vi "Get grpc_reflection_v1alpha_ListServiceResponse.vi"(8 "error in (no error)":errorcluster, 11 "gRPCid":T1) -> (0 "error out":errorcluster, 2 "package_templatemessage":T2, 3 "gRPCid out":T1)   [LabVIEW 2025, in "reflection_server.lvlib"]
uses:
  reflection_server.lvlib
  grpc_reflection_v1alpha_ListServiceResponse.ctl
  grpc_reflection_v1alpha_ServiceResponse.ctl
  <vilib>/gRPC/LabVIEW gRPC Library/Shared/grpcId.ctl
  grpc_reflection_v1alpha_ListServiceResponse_Flat.ctl
  grpc_reflection_v1alpha_ServiceResponse_Flat.ctl
  2ed25e12-861d-4677-8ead-ace2906b2041.vi
  <vilib>/gRPC/LabVIEW gRPC Library/Shared/TranslateGrpcError.vi
  FlatToRichgrpc_reflection_v1alpha_ServiceResponse.vi
  <vilib>/gRPC/LabVIEW gRPC Library/Server API/Server/Get Server DLL Path.vi
  <vilib>/Utility/error.llb/Error Cluster From Error Code.vi
  <vilib>/gRPC/LabVIEW gRPC Library/grpc-lvsupport-release.lvlib
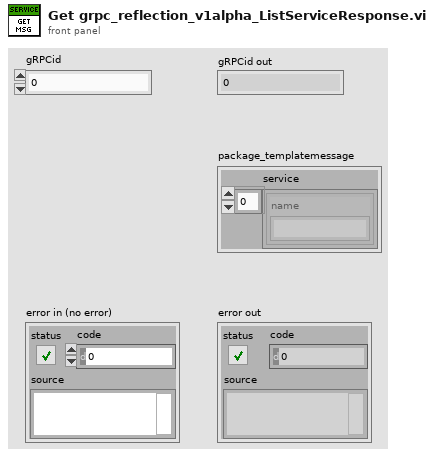
[diagram p1: front panel]
types:
  T1 = typedef "grpc-lvsupport-release.lvlib/grpcId.ctl" = u64
  T2 = typedef "reflection_server.lvlib/grpc_reflection_v1alpha_ListServiceResponse.ctl" = cluster{"service":T3[]}
  T3 = typedef "reflection_server.lvlib/grpc_reflection_v1alpha_ServiceResponse.ctl" = cluster{"name":string}
  T4 = typedef "reflection_server.lvlib/grpc_reflection_v1alpha_ListServiceResponse_Flat.ctl" = cluster{"service":T5[]}
  T5 = typedef "reflection_server.lvlib/grpc_reflection_v1alpha_ServiceResponse_Flat.ctl" = cluster{"name":string}
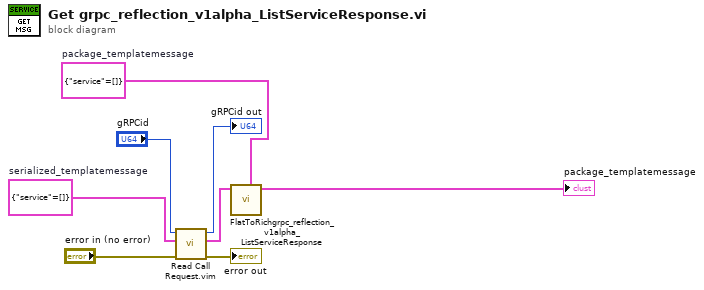
[diagram p0: block diagram]
diagram:
  w6 = T4 {"service"=[]}  # serialized_templatemessage
  w5 = T2 {"service"=[]}  # package_templatemessage
  n1 = call "Read Call Request.vim"("error in"="error in (no error)", "Request Type"=w6, "gRPCid in"="gRPCid") -> ("error out"=→"error out":errorcluster, "Request Data"=w4:T4, "gRPCid out"=→"gRPCid out":T1)  [unwired: 6 in]
  n2 = call "FlatToRichgrpc_reflection_v1alpha_ListServiceResponse.vi"("OutputClusterType"=w5, "InputCluster"=w4) -> ("OutputCluster"=→"package_templatemessage":T2)  [unwired: 9 in]
